vi "Ooi Wei Hong TP065329 Server.vi"() -> ()   [LabVIEW 2023]
uses:
  Control 2.ctl
  <vilib>/numeric/Random Number (Range) U64.vi
  <vilib>/numeric/sub_Random U32.vi
  <vilib>/Utility/file.llb/Write Delimited Spreadsheet (string).vi
  <vilib>/Utility/file.llb/Read Delimited Spreadsheet (string).vi
  <vilib>/regexp/Match Regular Expression.xnode
panel:
  in  "Tab Control":enum32{"Login", "Main", "Main 2"}(tab)
  in  "Username :":string
  in  "Password :":string
  in  "LoginBtn":bool
  in  "Next":bool
  in  "LogoutBtn":bool
  in  "Normal":cluster{u32, u32}[](array[cluster])
  in  "Bypass":cluster{u32, u32}[](array[cluster])
  in  "Alarm":cluster{u32, u32}[](array[cluster])
  in  "Tamper":cluster{u32, u32}[](array[cluster])
  out "Zone 1":bool
  out "Zone 2":bool caption="Zone 1"
  out "Zone 3":bool caption="Zone 1"
  out "Zone 4":bool caption="Zone 1"
  out "Zone 5":bool caption="Zone 1"
  out "Zone 6":bool caption="Zone 1"
  out "Current Time":timestamp
  out "Log":string[][](table)
  in  "Back":bool
  in  "LogoutBtn 2":bool
  in  "Logbook Table":path=path "Event_Logbook.csv"
  out "Passcode":dbl
  in  "Zone 6 Tamper":path=path "Sound/Zone 6 Tamper Detected.wav"
  in  "Zone 6 Bypass":path=path "Sound/Zone 6 Bypass Activated.wav"
  in  "Zone 6 Alarm":path=path "Sound/Zone 6 Security Breach Detected.wav"
  in  "Zone 5 Tamper":path=path "Sound/Zone 5 Tamper Detected.wav"
  in  "Zone 5 Bypass":path=path "Sound/Zone 5 Bypass Activated.wav"
  in  "Zone 5 Alarm":path=path "Sound/Zone 5 Security Breach Detected.wav"
  in  "Zone 4 Tamper":path=path "Sound/Zone 4 Tamper Detected.wav"
  in  "Zone 4 Bypass":path=path "Sound/Zone 4 Bypass Activated.wav"
  in  "Zone 4 Alarm":path=path "Sound/Zone 4 Security Breach Detected.wav"
  in  "Zone 3 Tamper":path=path "Sound/Zone 3 Tamper Detected.wav"
  in  "Zone 3 Bypass":path=path "Sound/Zone 3 Bypass Activated.wav"
  in  "Zone 3 Alarm":path=path "Sound/Zone 3 Security Breach Detected.wav"
  in  "Zone 2 Tamper":path=path "Sound/Zone 2 Tamper Detected.wav"
  in  "Zone 2 Bypass":path=path "Sound/Zone 2 Bypass Activated.wav"
  in  "Zone 2 Alarm":path=path "Sound/Zone 2 Security Breach Detected.wav"
  in  "Zone 1 Tamper":path=path "Sound/Zone 1 Tamper Detected.wav"
  in  "Zone 1 Bypass":path=path "Sound/Zone 1 Bypass Activated.wav"
  in  "Zone 1 Alarm":path=path "Sound/Zone 1 Security Breach Detected.wav"
  in  "File path (dialog if empty)":path=path "Users.txt"
  # "Vilantguard Technologies Security System"
  # "Security Surveillance Map"
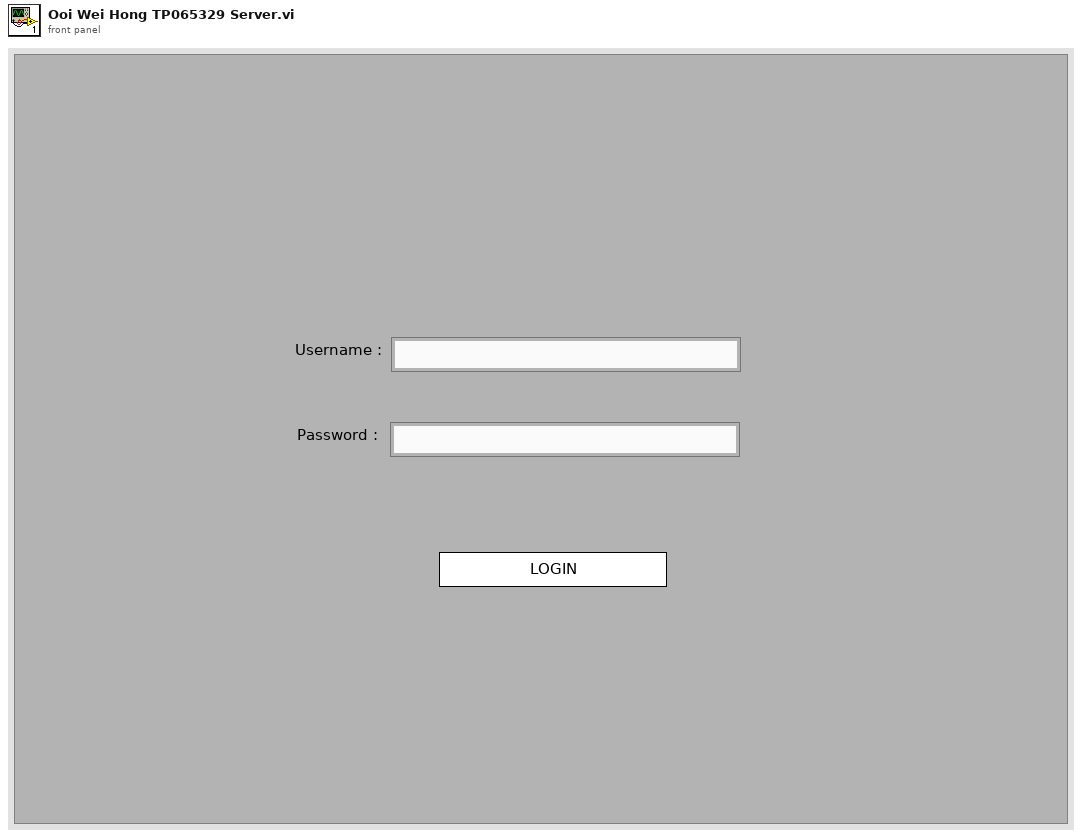
[diagram p1: front panel]
types:
  T1 = typedef "Control 2.ctl" = enum16{"Init", "Login", "Receive"}
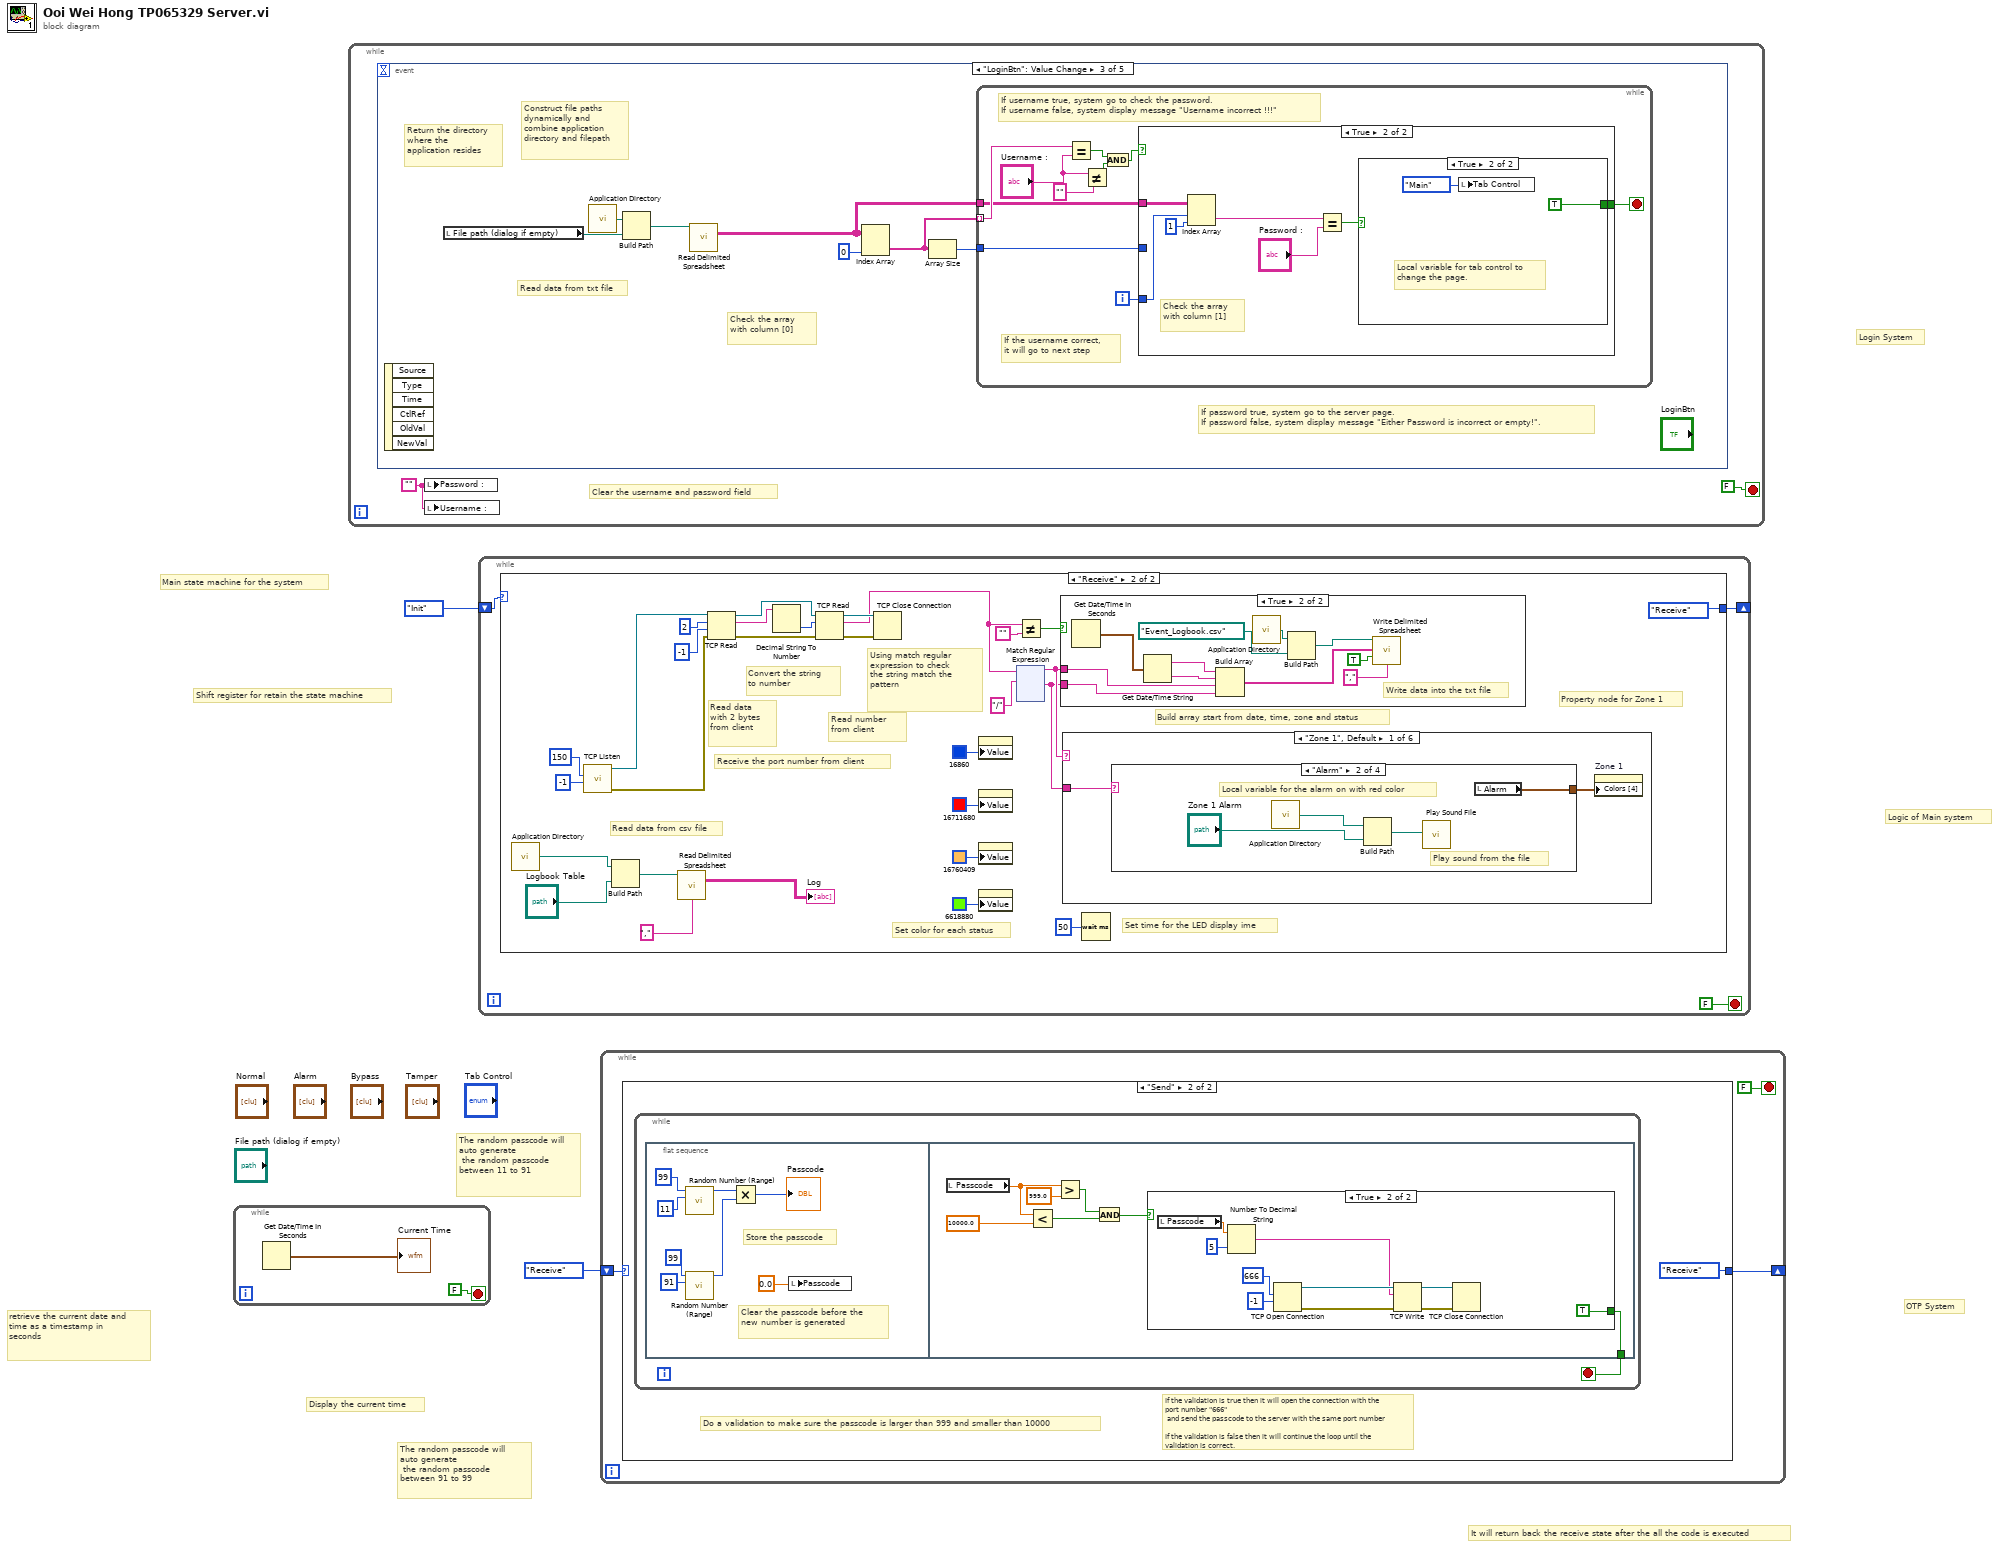
[diagram p0: block diagram]
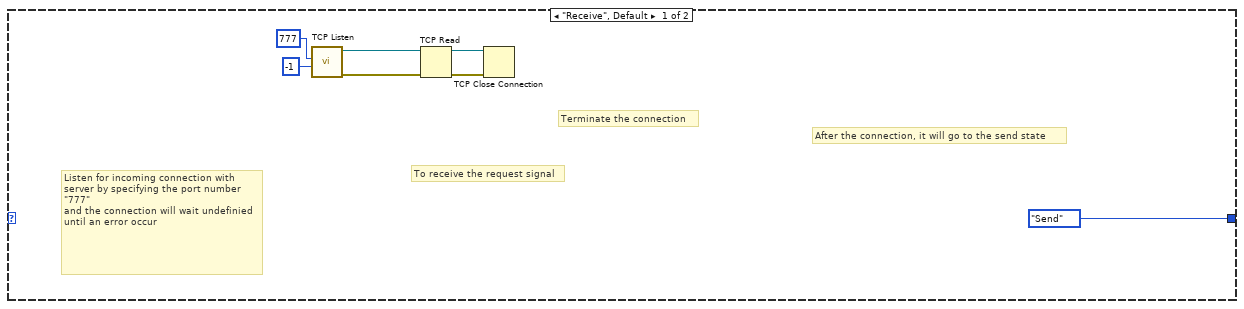
[diagram p2: hidden frame]
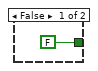
[diagram p3: hidden frame]
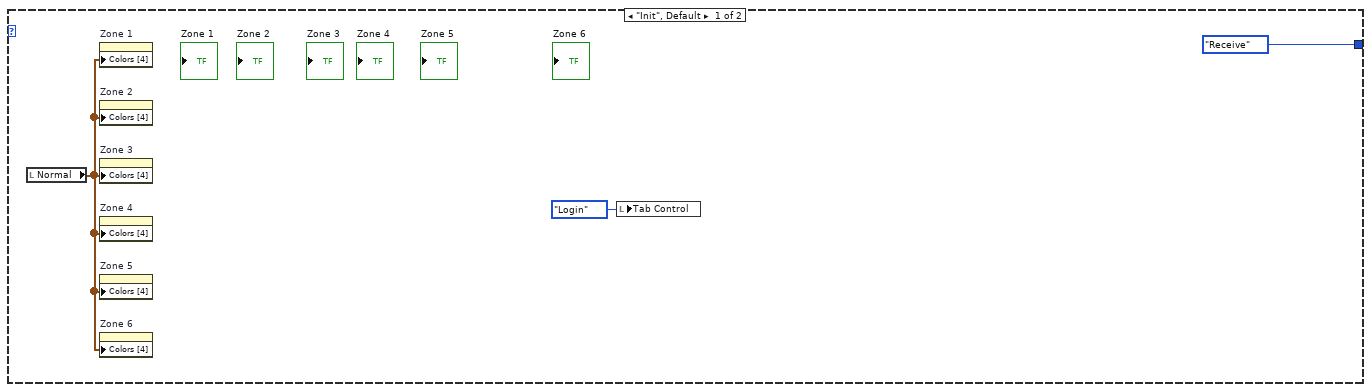
[diagram p4: hidden frame]
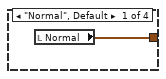
[diagram p6: hidden frame]
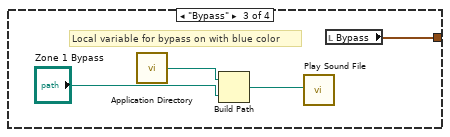
[diagram p7: hidden frame]
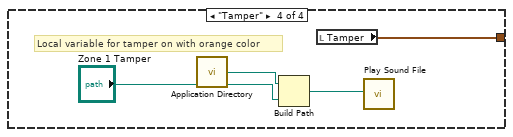
[diagram p8: hidden frame]
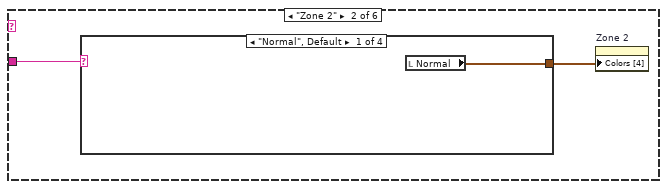
[diagram p9: hidden frame]
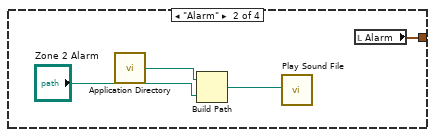
[diagram p10: hidden frame]
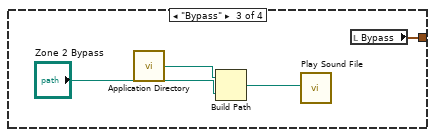
[diagram p11: hidden frame]
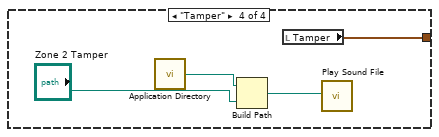
[diagram p12: hidden frame]
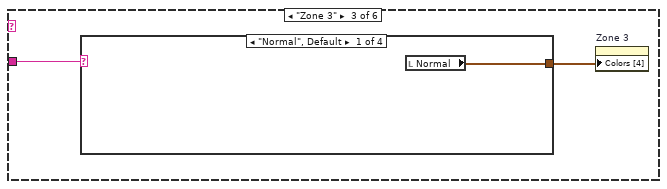
[diagram p13: hidden frame]
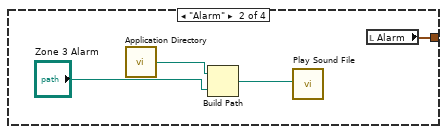
[diagram p14: hidden frame]
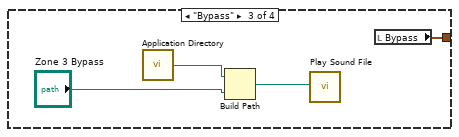
[diagram p15: hidden frame]
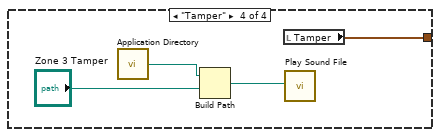
[diagram p16: hidden frame]
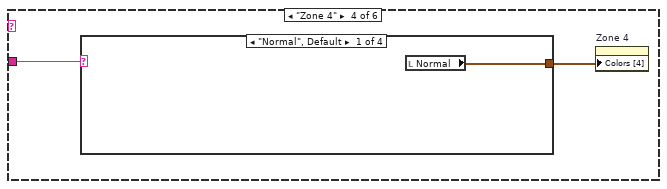
[diagram p17: hidden frame]
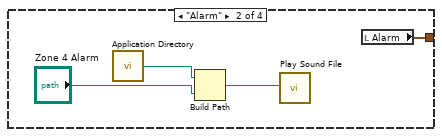
[diagram p18: hidden frame]
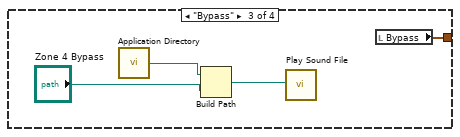
[diagram p19: hidden frame]
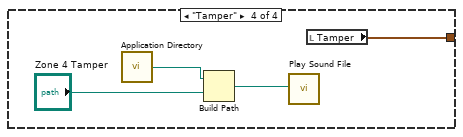
[diagram p20: hidden frame]
diagram:
  # "Shift register for retain the state machine"
  # "Main state machine for the system"
  # "Login System"
  # "Logic of Main system"
  # "OTP System"
  # "It will return back the receive state after the all the code is executed"
  # "The random passcode will auto generate\n the random passcode between 91 to 99"
  # "The random passcode will auto generate\n the random passcode between 11 to 91"
  # "Display the current time"
  # "retrieve the current date and time as a timestamp in seconds"
  n1 = while {
    stop <- FALSE stop-if-true
    n2 = Get Date/Time In Seconds() -> (seconds since 1Jan1904=→"Current Time":timestamp)
  }
  n3 = while {
    stop <- FALSE stop-if-true
    w5 = ""
    # "Clear the username and password field"
    n4 = event shown="[2] \"LoginBtn\": Value Change" {
      selector: _ -> [_ _ _ _ _]
      dyn-events: _ -> [_ _ _ _ _]
      timeout: _ -> [_ _ _ _ _]
      event Timeout {
        n5 = event-data() -> ()  [unwired: 1 in, 3 out]
      }
      event "Back": Value Change {
        n6 = event-data() -> ()  [unwired: 1 in, 6 out]
        n7 = local write "Tab Control"(enum32{"Login", "Main", "Main 2"}."Main" ("Tab Control")) -> ()
      }
      event "LoginBtn": Value Change {
        # "If password true, system go to the server page.\nIf password false, system display message \"Either Password is incorrect or empty!\"."
        # "Check the array with column [0]"
        # "Read data from txt file"
        # "Construct file paths dynamically and \ncombine application directory and filepath"
        # "Return the directory where the application resides"
        n8 = event-data() -> ()  [unwired: 1 in, 6 out]
        n9 = local read "File path (dialog if empty)"() -> (w12:path)
        n10 = call <vilib>:"Application Directory.vi"() -> ("Application Directory"=w14:path)
        n11 = Build Path(base path=w14, name or relative path=w12) -> (appended path=w13:path)
        n12 = call-poly <vilib>:"Read Delimited Spreadsheet.vi"("file path (dialog if empty)"=w13) -> ("all rows"=w8:string[][])  [unwired: 9 in, 5 out]
        n13 = Index Array "Index Array"(array=w8, index (col)=0 ("disabled index (col)")) -> (element=w10:string[])  [unwired: 1 in]
        n14 = Array Size(array=w10) -> (size(s)=w11:i32)
        n15 = while {
          tunnel: w10 -> [w24] mode=indexing
          tunnel: w8 -> [w22]
          tunnel: w11 -> [w21]
          i -> [w23]
          stop <- w20 stop-if-true
          # "If username true, system go to check the password.\nIf username false, system display message \"Username incorrect !!!\""
          # "If the username correct, \nit will go to next step"
          n16 = Equal?(x=w24, y="Username :") -> (x = y?=w16:bool)
          n17 = Not Equal?(x="Username :", y="") -> (x != y?=w15:bool)
          n18 = And(x=w16, y=w15) -> (x .and. y?=w17:bool)
          n19 = case shown="True" w17 {
            tunnel: w23 -> [w26 w35]
            tunnel: w22 -> [_ w34]
            tunnel: w21 -> [w29 _]
            tunnel: [w28 w30] -> w20
            frame False {
              # "Display \"Your username is incorrect! Please try again later...\" message"
              n20 = Decrement(x=w29) -> (x-1=w27:i32)
              n21 = Less?(x=w27, y=w26) -> (x < y?=w28:bool)
              n22 = Equal?(x=w27, y=w26) -> (x = y?=w25:bool)
              n23 = call "Display Message to User"("Enable"=w25) -> ()  [unwired: 9 in, 2 out]
            }
            frame True {
              # "Check the array with column [1]"
              n24 = Index Array "Index Array"(array=w34, index (row)=w35, index (col)=1) -> (element=w33:string)
              n25 = Equal?(x=w33, y="Password :") -> (x = y?=w31:bool)
              n26 = case shown="True" w31 {
                tunnel: [TRUE TRUE] -> w30
                frame False {
                  n27 = call "Display Message to User2"() -> ()  [unwired: 10 in, 2 out]
                }
                frame True {
                  # "Local variable for tab control to change the page."
                  n28 = local write "Tab Control"(enum32{"Login", "Main", "Main 2"}."Main" ("Tab Control")) -> ()
                }
              }
            }
          }
        }
      }
      event "LogoutBtn", "LogoutBtn 2": Value Change {
        n29 = event-data() -> ()  [unwired: 1 in, 6 out]
        n30 = local write "Tab Control"(enum32{"Login", "Main", "Main 2"}."Login" ("Tab Control")) -> ()
      }
      event "Next": Value Change {
        n31 = event-data() -> ()  [unwired: 1 in, 6 out]
        n32 = local write "Tab Control"(enum32{"Login", "Main", "Main 2"}."Main 2" ("Tab Control")) -> ()
      }
    }
    n33 = local write "Password :"(w5) -> ()
    n34 = local write "Username :"(w5) -> ()
  }
  n35 = while {
    shift-right: [w44] -> _
    shift-left: Control_2."Init" -> [w43]
    stop <- FALSE stop-if-true
    n36 = case shown="\"Receive\"" w43 {
      tunnel: [Control_2."Receive" Control_2."Receive"] -> w44
      frame "Init", Default {
        n37 = local read "Normal"() -> (w46:cluster{u32, u32}[])
        n38 = property on="Zone 1" class="Bool (strict)"("Colors [4]"=w46) -> ()  [unwired: 2 in, 2 out]
        n39 = property on="Zone 2" class="Bool (strict)"("Colors [4]"=w46) -> ()  [unwired: 2 in, 2 out]
        n40 = property on="Zone 3" class="Bool (strict)"("Colors [4]"=w46) -> ()  [unwired: 2 in, 2 out]
        n41 = property on="Zone 4" class="Bool (strict)"("Colors [4]"=w46) -> ()  [unwired: 2 in, 2 out]
        n42 = property on="Zone 5" class="Bool (strict)"("Colors [4]"=w46) -> ()  [unwired: 2 in, 2 out]
        n43 = property on="Zone 6" class="Bool (strict)"("Colors [4]"=w46) -> ()  [unwired: 2 in, 2 out]
        n44 = local write "Tab Control"(enum32{"Login", "Main", "Main 2"}."Login" ("Tab Control")) -> ()
      }
      frame "Receive" {
        # "Property node for Zone 1"
        # "Read data from csv file"
        # "Build array start from date, time, zone and status"
        # "Using match regular expression to check\nthe string match the pattern"
        # "Read number from client"
        # "Convert the string to number"
        # "Read data with 2 bytes from client"
        # "Receive the port number from client"
        # "Set time for the LED display ime"
        # "Set color for each status"
        n45 = call <vilib>:"Application Directory.vi"() -> ("Application Directory"=w51:path)
        n46 = call <vilib>:"TCP Listen.vi"("timeout ms (wait forever: -1)"=-1, "port"=u16 150) -> ("error out"=w66:errorcluster, "connection ID"=w63:refnum<k5>)  [unwired: 5 in, 3 out]
        n47 = Build Path(base path=w51, name or relative path="Logbook Table") -> (appended path=w50:path)
        n48 = call-poly <vilib>:"Read Delimited Spreadsheet.vi"("file path (dialog if empty)"=w50, "delimiter (\\t)"="," ("delimiter (\\t)")) -> ("all rows"=→"Log":string[][])  [unwired: 8 in, 5 out]
        n49 = TCP Read(connection ID=w63, bytes to read=2, error in (no error)=w66, 9:-1 ("timeout ms (25000)")) -> (connection ID out=w62:refnum<k5>, data out=w60:string, error out=w65:errorcluster)  [unwired: 1 in]
        n50 = Decimal String To Number(string=w60) -> (number=w59:i32)  [unwired: 2 in, 1 out]
        n51 = TCP Read(connection ID=w62, bytes to read=w59, error in (no error)=w65) -> (connection ID out=w61:refnum<k5>, data out=w57:string, error out=w64:errorcluster)  [unwired: 2 in]
        n52 = TCP Close Connection(connection ID=w61, error in (no error)=w64) -> ()  [unwired: 1 in, 2 out]
        n53 = property class="ColBox"("Value"=u32 16860) -> ()  [unwired: 2 in, 2 out]
        n54 = property class="ColBox"("Value"=u32 16711680) -> ()  [unwired: 2 in, 2 out]
        n55 = property class="ColBox"("Value"=u32 16760409) -> ()  [unwired: 2 in, 2 out]
        n56 = property class="ColBox"("Value"=u32 6618880) -> ()  [unwired: 2 in, 2 out]
        n57 = Not Equal?(x=w57, y="") -> (x != y?=w56:bool)
        n58 = xnode ("Match Regular Expression")("input string"=w57, "regular expression"="/") -> ("before match"=w54:string, "after match"=w53:string)  [unwired: 4 in, 3 out]
        n59 = case shown="True" w56 {
          tunnel: w54 -> [_ w84]
          tunnel: w53 -> [_ w83]
          frame False {
          }
          frame True {
            # "Write data into the txt file"
            n60 = Get Date/Time In Seconds() -> (seconds since 1Jan1904=w87:timestamp)
            n61 = Get Date/Time String(seconds (now)=w87) -> (date string=w86:string, time string=w85:string)  [unwired: 2 in]
            n62 = Build Array "Build Array"(w86, w85, w84, w83) -> (w79:string[])
            n63 = call <vilib>:"Application Directory.vi"() -> ("Application Directory"=w82:path)
            n64 = Build Path(base path=w82, name or relative path=path "Event_Logbook.csv") -> (appended path=w80:path)
            n65 = call-poly <vilib>:"Write Delimited Spreadsheet.vi"("file path (dialog if empty)"=w80, "1D data"=w79, "append to file? (new file:F)"=TRUE, "delimiter (\\t)"="," ("delimiter (\\t)")) -> ()  [unwired: 10 in, 2 out]
          }
        }
        n66 = case shown="\"Zone 1\", Default" w54 {
          tunnel: w53 -> [w205 w220 w235 w250 w265 w280]
          frame "Zone 1", Default {
            n67 = case shown="\"Alarm\"" w205 {
              tunnel: [w207 w211 w215 w219] -> w206
              frame "Normal", Default {
                n68 = local read "Normal"() -> (w207:cluster{u32, u32}[])
              }
              frame "Alarm" {
                # "Play sound from the file"
                # "Local variable for the alarm on with red color"
                n69 = call <vilib>:"Application Directory.vi"() -> ("Application Directory"=w210:path)
                n70 = Build Path(base path=w210, name or relative path="Zone 1 Alarm") -> (appended path=w209:path)
                n71 = call <vilib>:"Play Sound File.vi"("path"=w209) -> ()  [unwired: 9 in, 2 out]
                n72 = local read "Alarm"() -> (w211:cluster{u32, u32}[])
              }
              frame "Bypass" {
                # "Local variable for bypass on with blue color"
                n73 = call <vilib>:"Application Directory.vi"() -> ("Application Directory"=w214:path)
                n74 = Build Path(base path=w214, name or relative path="Zone 1 Bypass") -> (appended path=w213:path)
                n75 = call <vilib>:"Play Sound File.vi"("path"=w213) -> ()  [unwired: 9 in, 2 out]
                n76 = local read "Bypass"() -> (w215:cluster{u32, u32}[])
              }
              frame "Tamper" {
                # "Local variable for tamper on with orange color"
                n77 = call <vilib>:"Application Directory.vi"() -> ("Application Directory"=w218:path)
                n78 = Build Path(base path=w218, name or relative path="Zone 1 Tamper") -> (appended path=w217:path)
                n79 = local read "Tamper"() -> (w219:cluster{u32, u32}[])
                n80 = call <vilib>:"Play Sound File.vi"("path"=w217) -> ()  [unwired: 9 in, 2 out]
              }
            }
            n81 = property on="Zone 1" class="Bool (strict)"("Colors [4]"=w206) -> ()  [unwired: 2 in, 2 out]
          }
          frame "Zone 2" {
            n82 = case shown="\"Normal\", Default" w220 {
              tunnel: [w222 w226 w230 w234] -> w221
              frame "Normal", Default {
                n83 = local read "Normal"() -> (w222:cluster{u32, u32}[])
              }
              frame "Alarm" {
                n84 = call <vilib>:"Application Directory.vi"() -> ("Application Directory"=w225:path)
                n85 = Build Path(base path=w225, name or relative path="Zone 2 Alarm") -> (appended path=w224:path)
                n86 = call <vilib>:"Play Sound File.vi"("path"=w224) -> ()  [unwired: 9 in, 2 out]
                n87 = local read "Alarm"() -> (w226:cluster{u32, u32}[])
              }
              frame "Bypass" {
                n88 = call <vilib>:"Application Directory.vi"() -> ("Application Directory"=w229:path)
                n89 = Build Path(base path=w229, name or relative path="Zone 2 Bypass") -> (appended path=w228:path)
                n90 = call <vilib>:"Play Sound File.vi"("path"=w228) -> ()  [unwired: 9 in, 2 out]
                n91 = local read "Bypass"() -> (w230:cluster{u32, u32}[])
              }
              frame "Tamper" {
                n92 = call <vilib>:"Application Directory.vi"() -> ("Application Directory"=w233:path)
                n93 = Build Path(base path=w233, name or relative path="Zone 2 Tamper") -> (appended path=w232:path)
                n94 = local read "Tamper"() -> (w234:cluster{u32, u32}[])
                n95 = call <vilib>:"Play Sound File.vi"("path"=w232) -> ()  [unwired: 9 in, 2 out]
              }
            }
            n96 = property on="Zone 2" class="Bool (strict)"("Colors [4]"=w221) -> ()  [unwired: 2 in, 2 out]
          }
          frame "Zone 3" {
            n97 = case shown="\"Normal\", Default" w235 {
              tunnel: [w237 w241 w245 w249] -> w236
              frame "Normal", Default {
                n98 = local read "Normal"() -> (w237:cluster{u32, u32}[])
              }
              frame "Alarm" {
                n99 = call <vilib>:"Application Directory.vi"() -> ("Application Directory"=w240:path)
                n100 = Build Path(base path=w240, name or relative path="Zone 3 Alarm") -> (appended path=w239:path)
                n101 = call <vilib>:"Play Sound File.vi"("path"=w239) -> ()  [unwired: 9 in, 2 out]
                n102 = local read "Alarm"() -> (w241:cluster{u32, u32}[])
              }
              frame "Bypass" {
                n103 = call <vilib>:"Application Directory.vi"() -> ("Application Directory"=w243:path)
                n104 = Build Path(base path=w243, name or relative path="Zone 3 Bypass") -> (appended path=w242:path)
                n105 = call <vilib>:"Play Sound File.vi"("path"=w242) -> ()  [unwired: 9 in, 2 out]
                n106 = local read "Bypass"() -> (w245:cluster{u32, u32}[])
              }
              frame "Tamper" {
                n107 = call <vilib>:"Application Directory.vi"() -> ("Application Directory"=w246:path)
                n108 = Build Path(base path=w246, name or relative path="Zone 3 Tamper") -> (appended path=w247:path)
                n109 = local read "Tamper"() -> (w249:cluster{u32, u32}[])
                n110 = call <vilib>:"Play Sound File.vi"("path"=w247) -> ()  [unwired: 9 in, 2 out]
              }
            }
            n111 = property on="Zone 3" class="Bool (strict)"("Colors [4]"=w236) -> ()  [unwired: 2 in, 2 out]
          }
          frame "Zone 4" {
            n112 = case shown="\"Normal\", Default" w250 {
              tunnel: [w252 w256 w260 w264] -> w251
              frame "Normal", Default {
                n113 = local read "Normal"() -> (w252:cluster{u32, u32}[])
              }
              frame "Alarm" {
                n114 = call <vilib>:"Application Directory.vi"() -> ("Application Directory"=w253:path)
                n115 = Build Path(base path=w253, name or relative path="Zone 4 Alarm") -> (appended path=w254:path)
                n116 = call <vilib>:"Play Sound File.vi"("path"=w254) -> ()  [unwired: 9 in, 2 out]
                n117 = local read "Alarm"() -> (w256:cluster{u32, u32}[])
              }
              frame "Bypass" {
                n118 = call <vilib>:"Application Directory.vi"() -> ("Application Directory"=w258:path)
                n119 = Build Path(base path=w258, name or relative path="Zone 4 Bypass") -> (appended path=w257:path)
                n120 = call <vilib>:"Play Sound File.vi"("path"=w257) -> ()  [unwired: 9 in, 2 out]
                n121 = local read "Bypass"() -> (w260:cluster{u32, u32}[])
              }
              frame "Tamper" {
                n122 = call <vilib>:"Application Directory.vi"() -> ("Application Directory"=w261:path)
                n123 = Build Path(base path=w261, name or relative path="Zone 4 Tamper") -> (appended path=w262:path)
                n124 = call <vilib>:"Play Sound File.vi"("path"=w262) -> ()  [unwired: 9 in, 2 out]
                n125 = local read "Tamper"() -> (w264:cluster{u32, u32}[])
              }
            }
            n126 = property on="Zone 4" class="Bool (strict)"("Colors [4]"=w251) -> ()  [unwired: 2 in, 2 out]
          }
          frame "Zone 5" {
            n127 = case shown="\"Normal\", Default" w265 {
              tunnel: [w267 w271 w275 w279] -> w266
              frame "Normal", Default {
                n128 = local read "Normal"() -> (w267:cluster{u32, u32}[])
              }
              frame "Alarm" {
                n129 = call <vilib>:"Application Directory.vi"() -> ("Application Directory"=w269:path)
                n130 = Build Path(base path=w269, name or relative path="Zone 5 Alarm") -> (appended path=w268:path)
                n131 = call <vilib>:"Play Sound File.vi"("path"=w268) -> ()  [unwired: 9 in, 2 out]
                n132 = local read "Alarm"() -> (w271:cluster{u32, u32}[])
              }
              frame "Bypass" {
                n133 = call <vilib>:"Application Directory.vi"() -> ("Application Directory"=w273:path)
                n134 = Build Path(base path=w273, name or relative path="Zone 5 Bypass") -> (appended path=w272:path)
                n135 = call <vilib>:"Play Sound File.vi"("path"=w272) -> ()  [unwired: 9 in, 2 out]
                n136 = local read "Bypass"() -> (w275:cluster{u32, u32}[])
              }
              frame "Tamper" {
                n137 = call <vilib>:"Application Directory.vi"() -> ("Application Directory"=w276:path)
                n138 = Build Path(base path=w276, name or relative path="Zone 5 Tamper") -> (appended path=w277:path)
                n139 = call <vilib>:"Play Sound File.vi"("path"=w277) -> ()  [unwired: 9 in, 2 out]
                n140 = local read "Tamper"() -> (w279:cluster{u32, u32}[])
              }
            }
            n141 = property on="Zone 5" class="Bool (strict)"("Colors [4]"=w266) -> ()  [unwired: 2 in, 2 out]
          }
          frame "Zone 6" {
            n142 = case shown="\"Alarm\"" w280 {
              tunnel: [w282 w286 w290 w294] -> w281
              frame "Normal", Default {
                n143 = local read "Normal"() -> (w282:cluster{u32, u32}[])
              }
              frame "Alarm" {
                n144 = call <vilib>:"Application Directory.vi"() -> ("Application Directory"=w284:path)
                n145 = Build Path(base path=w284, name or relative path="Zone 6 Alarm") -> (appended path=w283:path)
                n146 = call <vilib>:"Play Sound File.vi"("path"=w283) -> ()  [unwired: 9 in, 2 out]
                n147 = local read "Alarm"() -> (w286:cluster{u32, u32}[])
              }
              frame "Bypass" {
                n148 = call <vilib>:"Application Directory.vi"() -> ("Application Directory"=w287:path)
                n149 = Build Path(base path=w287, name or relative path="Zone 6 Bypass") -> (appended path=w288:path)
                n150 = call <vilib>:"Play Sound File.vi"("path"=w288) -> ()  [unwired: 9 in, 2 out]
                n151 = local read "Bypass"() -> (w290:cluster{u32, u32}[])
              }
              frame "Tamper" {
                n152 = call <vilib>:"Application Directory.vi"() -> ("Application Directory"=w292:path)
                n153 = Build Path(base path=w292, name or relative path="Zone 6 Tamper") -> (appended path=w291:path)
                n154 = call <vilib>:"Play Sound File.vi"("path"=w291) -> ()  [unwired: 9 in, 2 out]
                n155 = local read "Tamper"() -> (w294:cluster{u32, u32}[])
              }
            }
            n156 = property on="Zone 6" class="Bool (strict)"("Colors [4]"=w281) -> ()  [unwired: 2 in, 2 out]
          }
        }
        n157 = Wait (ms)(milliseconds to wait=u32 50) -> ()  [unwired: 1 out]
      }
    }
  }
  n158 = while {
    shift-right: [w297] -> _
    shift-left: enum16{"Receive", "Send"}."Receive" -> [w296]
    stop <- FALSE stop-if-true
    n159 = case shown="\"Send\"" w296 {
      tunnel: [enum16{"Receive", "Send"}."Send" enum16{"Receive", "Send"}."Receive"] -> w297
      frame "Receive", Default {
        # "Terminate the connection"
        # "To receive the request signal"
        # "Listen for incoming connection with server by specifying the port number \"777\" \nand the connection will wait undefinied until an error occur"
        # "After the connection, it will go to the send state"
        n160 = call <vilib>:"TCP Listen.vi"("timeout ms (wait forever: -1)"=-1, "port"=u16 777) -> ("error out"=w302:errorcluster, "connection ID"=w304:refnum<k5>)  [unwired: 5 in, 3 out]
        n161 = TCP Read(connection ID=w304, error in (no error)=w302) -> (connection ID out=w303:refnum<k5>, error out=w301:errorcluster)  [unwired: 3 in, 1 out]
        n162 = TCP Close Connection(connection ID=w303, error in (no error)=w301) -> ()  [unwired: 1 in, 2 out]
      }
      frame "Send" {
        # "If the validation is true then it will open the connection with the port number \"666\"\n and send the passcode to the server with the same port number\n\nIf the validation is false then it will continue the loop until the validation is correct."
        # "Do a validation to make sure the passcode is larger than 999 and smaller than 10000"
        n163 = while {
          stop <- w306 stop-if-true
          n164 = flat-sequence {
            tunnel: [w315] -> w306
            frame #0 {
              # "Clear the passcode before the new number is generated"
              # "Store the passcode"
              n165 = call-poly <vilib>:"Random Number (Range).vi"("lower bound (0)"=u64 11, "upper bound (100)"=u64 99) -> ("number"=w313:u64)  [unwired: 9 in]
              n166 = call-poly <vilib>:"Random Number (Range).vi"("lower bound (0)"=u64 91, "upper bound (100)"=u64 99) -> ("number"=w314:u64)  [unwired: 9 in]
              n167 = Multiply(x=w313, y=w314) -> (x*y=→"Passcode":u64)
              n168 = local write "Passcode"(0.0 ("x*y")) -> ()
            }
            frame #1 {
              n169 = local read "Passcode"() -> (w320:dbl)
              n170 = Less?(x=w320, y=10000.0) -> (x < y?=w321:bool)
              n171 = Greater?(x=w320, y=999.0) -> (0:w318:bool)
              n172 = And(x=w318, y=w321) -> (x .and. y?=w319:bool)
              n173 = case shown="True" w319 {
                tunnel: [FALSE TRUE] -> w315
                frame False {
                }
                frame True {
                  n174 = local read "Passcode"() -> (w326:dbl)
                  n175 = Number To Decimal String(number=w326, width (-)=i16 5) -> (decimal integer string=w324:string)
                  n176 = TCP Open Connection(remote port or service name=u16 666, timeout ms (60000)=-1) -> (connection ID=w332:refnum<k5>, error out=w329:errorcluster)  [unwired: 3 in]
                  n177 = TCP Write(connection ID=w332, data in=w324, error in (no error)=w329) -> (connection ID out=w331:refnum<k5>, error out=w330:errorcluster)  [unwired: 1 in, 1 out]
                  n178 = TCP Close Connection(connection ID=w331, error in (no error)=w330) -> ()  [unwired: 1 in, 2 out]
                }
              }
            }
          }
        }
      }
    }
  }
